vi "sample-profiled-pid-turn-to-angle.vi"() -> ()   [LabVIEW 2019]
uses:
  <vilib>/Rock Robotics/WPI/ThirdParty/JAS_Junk/TrajLib/TrapProfState_New.vi
  <vilib>/Rock Robotics/WPI/ThirdParty/JAS_Junk/TrajLib/PIDController_NewPeriod.vi
  <vilib>/Rock Robotics/SystemInterfaces/NetworkCommunication/NetComm_UsageReport_report.vi
  <vilib>/Rock Robotics/WPI/ThirdParty/JAS_Junk/TrajLib/PIDController_SetIntegratorRange.vi
  <vilib>/Rock Robotics/WPI/ThirdParty/JAS_Junk/TrajLib/PIDController_EnableContinousInput.vi
  <vilib>/Rock Robotics/WPI/ThirdParty/JAS_Junk/TrajLib/PIDController_SetTolerancePandV.vi
  <vilib>/Rock Robotics/WPI/ThirdParty/JAS_Junk/TrajLib/ProfiledPIDController_Reset.vi
  <vilib>/Rock Robotics/WPI/ThirdParty/JAS_Junk/TrajLib/LinearFilter_ResetToValue.vi
  <vilib>/Rock Robotics/WPI/ThirdParty/JAS_Junk/TrajLib/LinearFilter_Calculate.vi
  <vilib>/Rock Robotics/WPI/ThirdParty/JAS_Junk/TrajLib/ProfiledPIDController_SetGoal_PosOnly.vi
  <vilib>/Rock Robotics/WPI/ThirdParty/JAS_Junk/TrajLib/ProfiledPIDController_Calculate_Meas.vi
  <vilib>/Rock Robotics/WPI/ThirdParty/JAS_Junk/TrajLib/PIDController_GetVelocityError.vi
  <vilib>/Rock Robotics/WPI/ThirdParty/JAS_Junk/TrajLib/PIDController_GetPositionError.vi
  <vilib>/Rock Robotics/WPI/ThirdParty/JAS_Junk/TrajLib/PIDController_AtSetpoint.vi
  <vilib>/Rock Robotics/WPI/ThirdParty/JAS_Junk/TrajLib/TrapProfState_Equals.vi
  <vilib>/Rock Robotics/WPI/ThirdParty/JAS_Junk/TrajLib/PIDController_Reset.vi
  <vilib>/Rock Robotics/WPI/ThirdParty/JAS_Junk/TrajLib/ProfiledPIDController_SetGoal.vi
  <vilib>/Rock Robotics/WPI/ThirdParty/JAS_Junk/TrajLib/PIDController_Calculate_SP_PV.vi
  <vilib>/Rock Robotics/WPI/ThirdParty/JAS_Junk/TrajLib/TrapProfile_New.vi
  <vilib>/Rock Robotics/WPI/ThirdParty/JAS_Junk/TrajLib/ProfiledPIDController_GetPeriod.vi
  <vilib>/Rock Robotics/WPI/ThirdParty/JAS_Junk/TrajLib/TrapProfile_Calculate.vi
  <vilib>/Rock Robotics/WPI/ThirdParty/JAS_Junk/TrajLib/ControllerUtil_GetModulusError.vi
  <vilib>/Rock Robotics/WPI/ThirdParty/JAS_Junk/TrajLib/PIDController_SetSetpoint.vi
  <vilib>/Rock Robotics/WPI/ThirdParty/JAS_Junk/TrajLib/PIDController_Calculate_PV.vi
  <vilib>/Rock Robotics/WPI/ThirdParty/JAS_Junk/TrajLib/TrapProfile_ShouldFlipAcceleration.vi
  <vilib>/Rock Robotics/WPI/ThirdParty/JAS_Junk/TrajLib/TrapProfile_Direct.vi
  <vilib>/Rock Robotics/WPI/ThirdParty/JAS_Junk/TrajLib/PIDController_GetPeriod.vi
  <vilib>/Rock Robotics/WPI/ThirdParty/JAS_Junk/TrajLib/Util_LibraryGlobals.vi
  <vilib>/Rock Robotics/WPI/ThirdParty/JAS_Junk/TrajLib/LinearFilter_MovingAverage.vi
  <vilib>/Rock Robotics/WPI/ThirdParty/JAS_Junk/TrajLib/LinearFilter_LowPassBW1.vi
  <vilib>/Rock Robotics/WPI/ThirdParty/JAS_Junk/TrajLib/LinearFilter_LowPassBW2.vi
  <vilib>/Rock Robotics/WPI/ThirdParty/JAS_Junk/TrajLib/LinearFilter_HighPassBW1.vi
  <vilib>/Rock Robotics/WPI/ThirdParty/JAS_Junk/TrajLib/LinearFilter_HighPassBW2.vi
  <vilib>/Rock Robotics/WPI/ThirdParty/JAS_Junk/TrajLib/Trajectory_Library.lvlib
  <vilib>/ptbypt/NI_PtbyPt.lvlib
panel:
  in  "Tab Control":enum32{"Operation", "Tuning"}(tab)
  out "Targets along the way":T1(graph)
  in  "SP - Desired Angle\n (Deg)":dbl(slide) scale=-10.0..350.0
  out "PV - Current Angle\n (Deg)":dbl(slide) scale=-10.0..350.0
  out "Goal":T2(graph)
  out "Motor Output":dbl format="%13.3f"
  out "AtSetpoint":bool
  out "AtGoal":bool
  out "PositionError  (Deg)":dbl format="%13.2f"
  out "VelocityError  (Deg/Sec)":dbl format="%13.2f"
  out "Velocity  (Deg/Sec)":dbl format="%13.2f"
  in  "Kp":dbl=0.08 format="%#_13g"
  in  "Ki":dbl=0.15 format="%#_13g"
  in  "Kd":dbl format="%#_13g"
  in  "Minimum Integral":dbl=-0.3 format="%#_13g"
  in  "Maximum Integral":dbl=0.3 format="%#_13g"
  in  "Max Speed   (Deg/Sec)":dbl=30.0 format="%#_13g"
  in  "Max Accel  (Deg/Sec^2)":dbl=5.0 format="%#_13g"
  in  "PositionTolerance\n(Deg)":dbl=1.0 format="%#_13g"
  in  "VelocityTolerance\n(Deg/Sec)":dbl=0.05 format="%#_13g"
  # "SET THESE BEFORE EXECUTING THIS PROGRAM."
  # "PID Tuning Parameters"
  # "Desired Profile Performance"
  # "Desired On Target Tolerance"
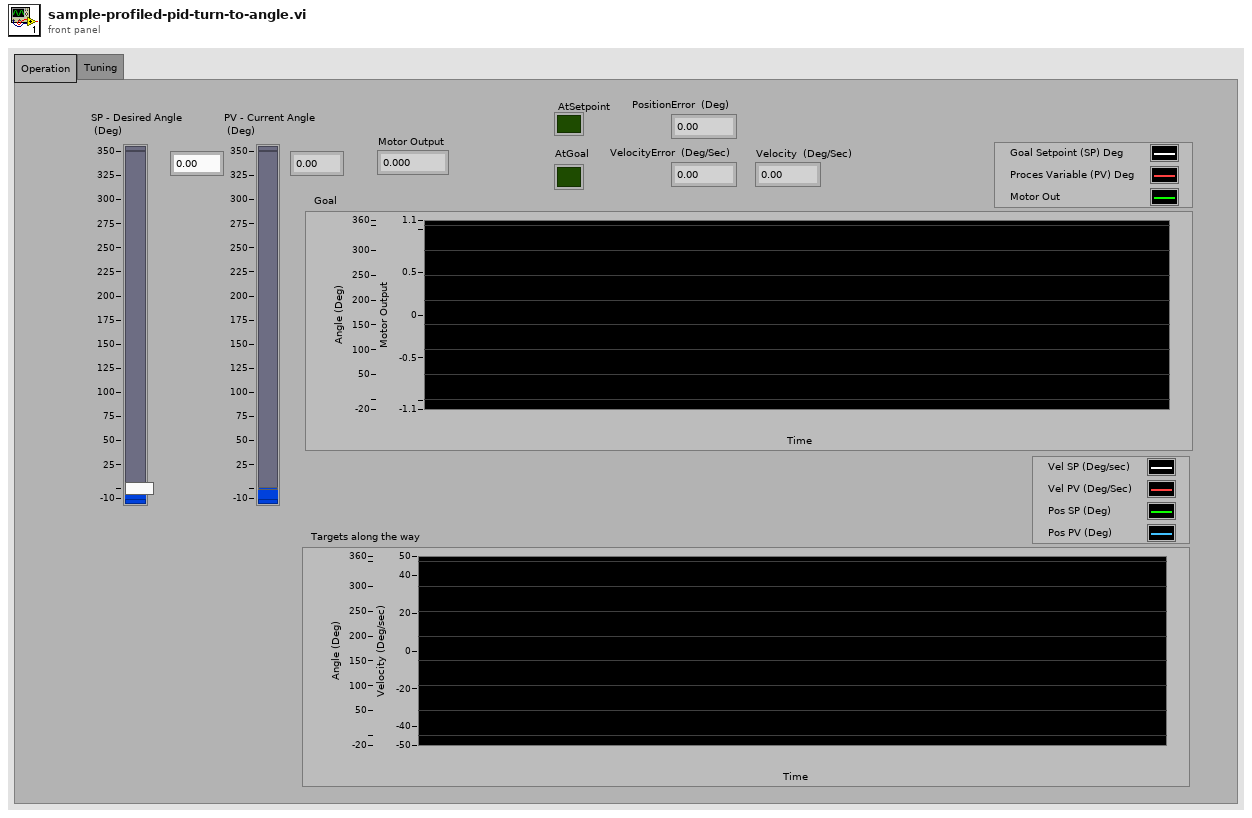
[diagram p1: front panel]
types:
  T1 = cluster{"SP - Desired Heading\n (Deg)":dbl, "PV - Current Heading\n (Deg)":dbl, "upper limit":dbl, dbl}
  T2 = cluster{"SP - Desired Position\n (Inch)":dbl, "upper limit":dbl, "upper limit":dbl}
  T3 = typedef "Trajectory_Library.lvlib/TRAPEZOID_PROFILE_CONSTRAINT.ctl" = cluster{"MaxVelocity":dbl, "MaxAcceleration":dbl}
  T4 = typedef "Trajectory_Library.lvlib/PROFILED_PID_CONTROLLER.ctl" = cluster{"Controller":T5, "Goal":T6, "Setpoint":T6, "Constraint":T3}
  T5 = typedef "Trajectory_Library.lvlib/PID_CONTROLLER.ctl" = cluster{"Kp":dbl, "Ki":dbl, "Kd":dbl, "Period":dbl, "Max_Integral":dbl, "Min_Integral":dbl, "Max_Input":dbl, "Min_Input":dbl, "Continuous":bool, "PositionError":dbl, "VelocityError":dbl, "PrevError":dbl, "TotalError":dbl, "PositionTolerance":dbl, "VelocityTolerance":dbl, "SetPoint":dbl, "Kf":dbl, "Prev_Deriv":dbl, "Prev_Deriv 2":dbl, "DerivativeFilter":bool, "Min_Output":dbl, "Max_Output":dbl, "Prev_F_P":dbl, "Prev_F_P_2":dbl, "AntiWindupActive":bool, "Measurement":dbl}
  T6 = typedef "Trajectory_Library.lvlib/TRAPEZOID_PROFILE_STATE.ctl" = cluster{"Position":dbl, "Velocity":dbl}
  T7 = enum16{"Moving Average", "Low Pass 1st Order Butterworth", "Low Pass 2nd Order Butterworth", "High Pass 1st Order Butterworth", "High Pass 2nd Order Butterworth"}
  T8 = cluster{"SP - Desired Angle\n (Deg)":dbl, "modulus":dbl, "upper limit":dbl}
  T9 = cluster{"Velocity":dbl, dbl, "Position":dbl, "modulus":dbl}
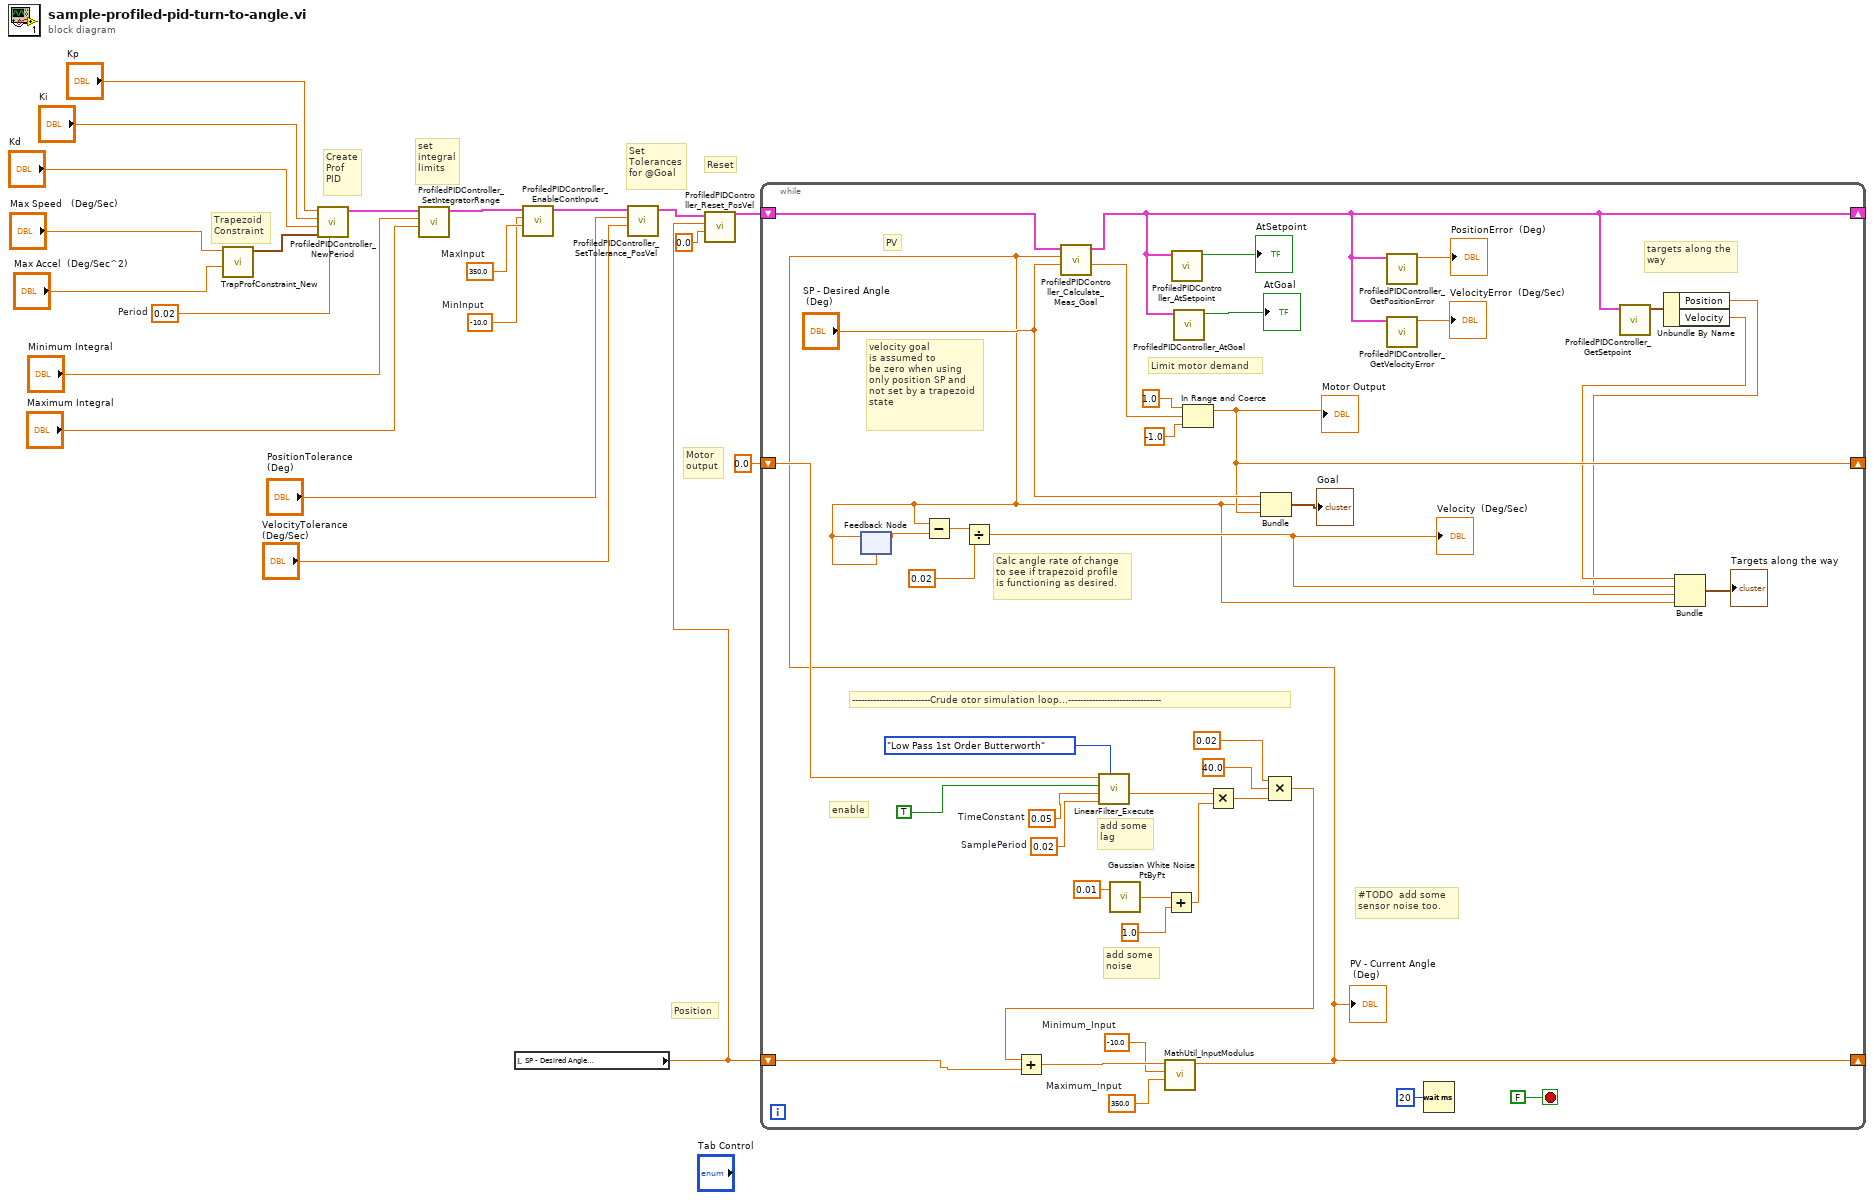
[diagram p0: block diagram]
diagram:
  w1 = -10.0  # MinInput
  w2 = 350.0  # MaxInput
  w18 = 0.02  # Period
  # "Reset"
  # "Position"
  # "Motor\noutput"
  # "set\nintegral\nlimits"
  # "Trapezoid\nConstraint"
  # "Set\nTolerances\nfor @Goal"
  # "Create\nProf\nPID"
  n1 = call <vilib>:"TrapProfConstraint_New.vi"("Max Accel"="Max Accel  (Deg/Sec^2)", "Max Speed (M/S)"="Max Speed   (Deg/Sec)") -> ("TRAPEZOID_PROFILE_CONSTRAINT"=w21:T3)  [unwired: 9 in]
  n2 = call <vilib>:"ProfiledPIDController_NewPeriod.vi"("Period"=w18, "Constraints"=w21, "Kd"="Kd", "Ki"="Ki", "Kp"="Kp") -> ("PROFILED_PID_CONTROLLER"=w12:T4)  [unwired: 6 in]
  n3 = call <vilib>:"ProfiledPIDController_SetIntegratorRange.vi"("Maximum"="Maximum Integral", "Minimum"="Minimum Integral", "in PROFILED_PID_CONTROLLER"=w12) -> ("out PROFILED_PID_CONTROLLER"=w4:T4)  [unwired: 8 in]
  n4 = local read "SP - Desired Angle\n (Deg)"() -> (w5:dbl)
  n5 = call <vilib>:"ProfiledPIDController_EnableContInput.vi"("MaxInput"=w2, "MinInput"=w1, "in PROFILED_PID_CONTROLLER"=w4) -> ("out PROFILED_PID_CONTROLLER"=w3:T4)  [unwired: 8 in]
  n6 = call <vilib>:"ProfiledPIDController_SetTolerance_PosVel.vi"("VelocityTolerance"="VelocityTolerance\n(Deg/Sec)", "PositionTolerance"="PositionTolerance\n(Deg)", "in PROFILED_PID_CONTROLLER"=w3) -> ("out PROFILED_PID_CONTROLLER"=w7:T4)  [unwired: 8 in]
  n7 = call <vilib>:"ProfiledPIDController_Reset_PosVel.vi"("Velocity"=0.0, "Position"=w5, "in PROFILED_PID_CONTROLLER"=w7) -> ("out PROFILED_PID_CONTROLLER"=w8:T4)  [unwired: 8 in]
  n8 = while {
    shift-right: [w30] -> _
    shift-left: w8 -> [w62]
    shift-right: [w24] -> _
    shift-left: w5 -> [w35]
    shift-right: [w34] -> _
    shift-left: 0.0 ("upper limit") -> [w33]
    stop <- FALSE stop-if-true
    w22 = -10.0  # Minimum_Input
    w23 = 350.0  # Maximum_Input
    w37 = 0.02  # SamplePeriod
    w36 = 0.05  # TimeConstant
    # "Limit motor demand"
    # "targets along the\nway"
    # "enable"
    # "PV"
    # "#TODO  add some\nsensor noise too."
    # "add some\nnoise"
    # "add some\nlag"
    # "--------------------------Crude otor simulation loop...-------------------------------"
    # "Calc angle rate of change\nto see if trapezoid profile\nis functioning as desired."
    # "velocity goal\nis assumed to \nbe zero when using\nonly position SP and\nnot set by a trapezoid\nstate"
    n9 = call <vilib>:"LinearFilter_Execute.vi"("Filter Type"=T7."Low Pass 1st Order Butterworth", "SamplePeriod"=w37, "TimeConstant"=w36, "Enable"=TRUE, "Input"=w33) -> ("Output"=w44:dbl)  [unwired: 5 in, 1 out]
    n10 = call <vilib>:"Gaussian White Noise PtByPt.vi"("standard deviation"=0.01) -> ("Gaussian white noise"=w43:dbl)  [unwired: 2 in]
    n11 = Add(x=w43, y=1.0) -> (x+y=w45:dbl)
    n12 = Multiply(x=w44, y=w45) -> (x*y=w46:dbl)
    n13 = Compound Arithmetic op=MULTIPLY(0.02 ("value"), 40.0 ("value"), w46) -> (w47:dbl)
    n14 = Add(x=w47, y=w35) -> (x+y=w25:dbl)
    n15 = call <vilib>:"MathUtil_InputModulus.vi"("Maximum_Input"=w23, "Minimum_Input"=w22, "Input"=w25) -> ("modulus"=w24:dbl)  [unwired: 8 in]
    "PV - Current Angle\n (Deg)" <- w24
    n16 = feedback-in #1(w24) -> ()
    n17 = feedback #1(w24) -> (w54:dbl)
    n18 = Subtract(x=w24, y=w54) -> (x-y=w53:dbl)
    n19 = Divide(x=w53, y=0.02) -> (x/y=w27:dbl)
    "Velocity  (Deg/Sec)" <- w27
    n20 = call <vilib>:"ProfiledPIDController_Calculate_Meas_Goal.vi"("SP-Goal"="SP - Desired Angle\n (Deg)", "PV-Measurement"=w24, "in PROFILED_PID_CONTROLLER"=w62) -> ("CO-ControlOutput"=w55:dbl, "out PROFILED_PID_CONTROLLER"=w30:T4)  [unwired: 7 in]
    n21 = call <vilib>:"ProfiledPIDController_AtSetpoint.vi"("in PROFILED_PID_CONTROLLER"=w30) -> ("AtSetpoint"=→"AtSetpoint":bool)  [unwired: 10 in]
    n22 = call <vilib>:"ProfiledPIDController_AtGoal.vi"("in PROFILED_PID_CONTROLLER"=w30) -> ("AtGoal"=→"AtGoal":bool)  [unwired: 10 in]
    n23 = In Range and Coerce(upper limit=1.0, x=w55, lower limit=-1.0) -> (coerced(x)=w34:dbl)  [unwired: 1 out]
    "Motor Output" <- w34
    n24 = Bundle("SP - Desired Angle\n (Deg)"="SP - Desired Angle\n (Deg)", "modulus"=w24, "upper limit"=w34) -> (→"Goal":T8)  [unwired: 1 in]
    n25 = call <vilib>:"ProfiledPIDController_GetPositionError.vi"("in PROFILED_PID_CONTROLLER"=w30) -> ("PositionError"=→"PositionError  (Deg)":dbl)  [unwired: 10 in]
    n26 = call <vilib>:"ProfiledPIDController_GetVelocityError.vi"("in PROFILED_PID_CONTROLLER"=w30) -> ("VelocityError"=→"VelocityError  (Deg/Sec)":dbl)  [unwired: 10 in]
    n27 = Wait (ms)(milliseconds to wait=u32 20) -> ()  [unwired: 1 out]
    n28 = call <vilib>:"ProfiledPIDController_GetSetpoint.vi"("in PROFILED_PID_CONTROLLER"=w30) -> ("Setpoint"=w29:T6)  [unwired: 10 in]
    n29 = Unbundle By Name(w29) -> ("Position"=w26:dbl, "Velocity"=w28:dbl)
    n30 = Bundle("Velocity"=w28, w27, "Position"=w26, "modulus"=w24) -> (→"Targets along the way":T9)  [unwired: 1 in]
  }
